vi "Initialize.vi"(7 "3D Picture Refnum":refnum<vi>, 8 "error in":errorcluster, 11 "AR Example.lvlib:UI.lvclass":refnum<class "UI.lvclass">) -> (0 "error out":errorcluster, 3 "App out":refnum<class "App.lvclass">)   [LabVIEW 2020, in "AR Example.lvlib" / "App.lvclass"]
uses:
  App.lvclass
  UI/UI.lvclass
  UI/Tab Control.ctl
  App.lvclass/App.ctl
  g_ar_toolkit.image/CreateEmptyImageARGB.vi
  g_ar_toolkit.image/CreateEmptyImageARGB.vi/3321fa97-f432-4e1e-8db9-a0df79aed21b.vi
  g_ar_toolkit.image/ARGBColourToU32.vi
  g_ar_toolkit.common/Module Path.vi
  <vilib>/Utility/error.llb/Error Cluster From Error Code.vi
  g_ar_toolkit.image/g_ar_toolkit.image.lvlib
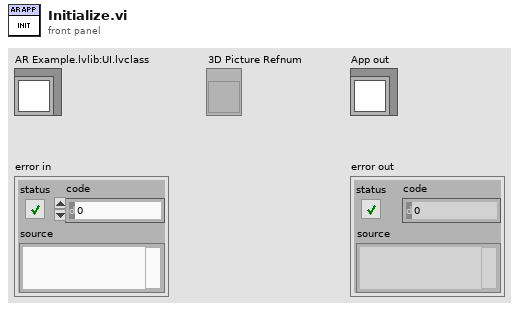
[diagram p1: front panel]
types:
  T1 = typedef "AR Example.lvlib/UI.lvclass/Tab Control.ctl" = enum8{"Config Load", "Camera Selection", "Camera Calibration"}
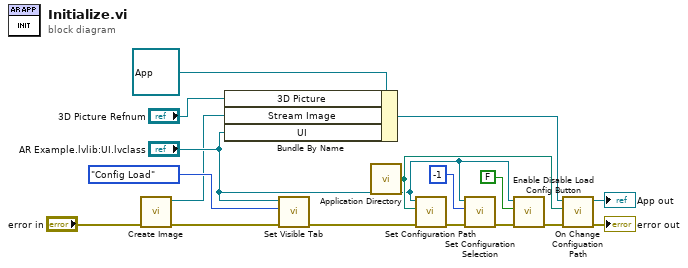
[diagram p0: block diagram]
diagram:
  n1 = call-poly "Create Image.vi"("error in (no error)"="error in") -> ("error out"=w3:errorcluster, "New ARGB Image"=w2:refnum<data-value>)  [unwired: 9 in]
  n2 = Bundle By Name(cluster=refnum<class "App.lvclass"> refnum ("App out"), "3D Picture"="3D Picture Refnum", "Stream Image"=w2, "UI"="AR Example.lvlib:UI.lvclass") -> (w13:refnum<class "App.lvclass">)
  n3 = call-dynamic "Set Visible Tab.vi"("error in (no error)"=w3, "Value"=Tab_Control."Config Load", "UI in"="AR Example.lvlib:UI.lvclass") -> ("error out"=w8:errorcluster)  [unwired: 8 in]
  n4 = call <vilib>:"Application Directory.vi"() -> ("Application Directory"=w6:path)
  n5 = call-dynamic "Set Configuration Path.vi"("error in (no error)"=w8, "Value"=w6, "UI in"="AR Example.lvlib:UI.lvclass") -> ("error out"=w16:errorcluster)  [unwired: 8 in]
  n6 = call-dynamic "Set Configuration Selection.vi"("error in (no error)"=w16, "Selection"=-1, "UI in"="AR Example.lvlib:UI.lvclass") -> ("error out"=w14:errorcluster)  [unwired: 8 in]
  n7 = call-dynamic "Enable Disable Load Config Button.vi"("error in (no error)"=w14, "Enable?"=FALSE, "UI in"="AR Example.lvlib:UI.lvclass") -> ("error out"=w10:errorcluster)  [unwired: 8 in]
  n8 = call "On Change Configuation Path.vi"("error in (no error)"=w10, "Path"=w6, "App in"=w13) -> ("error out"=→"error out":errorcluster, "App out"=→"App out":refnum<class "App.lvclass">)  [unwired: 7 in]
